vi "Interpret ADS Packet.vi"(8 "Error In":errorcluster, 11 "ADS Packet":string) -> (0 "Error Out":errorcluster, 2 "AMS":T1, 3 "Data":u8[](array[numeric]), 4 "Invoke ID":u32, 5 "State Flag":T3=4 items=["TCP Request"=4, "TCP Response"=5, "UDP Request"=68, "UDP Respone"=69], 6 "ADS Error":T2 items=["NoError"=0, "InternalError"=1, "NoRTime"=2, "LockedMemoryError"=3, "MailBoxError"=4, "WrongHMsg"=5, "TargetPortNotFound"=6, "TargetMachineNotFound"=7, "UnknownCommandID"=8, "BadTaskID"=9, "NoIO"=10, "UnknownAmsCommand"=11, "Win32Error"=12, "PortNotConnected"=13, "InvalidAmsLength"=14, "InvalidAmsNetID"=15, "AmsSyncAmsError"=22, "AmsSyncNoIndexMap"=23, "InvalidAmsPort"=24, "NoMemory"=25, "TCPSendError"=26, "HostUnreachable"=27, "NoLockedMemory"=1280, "MailboxFull"=1282, "DeviceError"=1792, "DeviceServiceNotSupported"=1793, "DeviceInvalidGroup"=1794, "DeviceInvalidOffset"=1795, "DeviceInvalidAccess"=1796, "DeviceInvalidSize"=1797, "DeviceInvalidData"=1798, "DeviceNotReady"=1799, "DeviceBusy"=1800, "DeviceInvalidContext"=1801, "DeviceNoMemory"=1802, "DeviceInvalidParam"=1803, "DeviceNotFound"=1804, "DeviceSyntaxError"=1805, "DeviceIncompatible"=1806, "DeviceExists"=1807, "DeviceSymbolNotFound"=1808, "DeviceSymbolVersionInvalid"=1809, "DeviceInvalidState"=1810, "DeviceTransModeNotSupported"=1811, "DeviceNotifyHandleInvalid"=1812, "DeviceClientUnknown"=1813, "DeviceNoMoreHandles"=1814, "DeviceInvalidWatchsize"=1815, "DeviceNotInitialized"=1816, "DeviceTimeOut"=1817, "DeviceNoInterface"=1818, "DeviceInvalidInterface"=1819, "DeviceInvalidCLSID"=1820, "DeviceInvalidObjectID"=1821, "ClientError"=1856, "ClientInvalidParameter"=1857, "ClientListEmpty"=1858, "ClientVariableInUse"=1859, "ClientDuplicateInvokeID"=1860, "ClientSyncTimeOut"=1861, "ClientW32OR"=1862, "ClientTimeoutInvalid"=1863, "ClientPortNotOpen"=1864, "ClientNoAmsAddr"=1865, "ClientSyncInternal"=1872, "ClientAddHash"=1873, "ClientRemoveHash"=1874, "ClientNoMoreSymbols"=1875, "ClientSyncResInvalid"=1876, "ClientSyncPortLocked"=1877, "ClientQueueFull"=1878], 7 "Command ID":T4=enum."ADS Read Device Info")   [LabVIEW 2019, in "TwinCAT ADS.lvlib"]
uses:
  <userlib>/PMA/TwinCAT ADS.lvlib
  <userlib>/PMA/Low Level/TypeDefs/Command Id.ctl
  <userlib>/PMA/Low Level/TypeDefs/State Flag.ctl
  <userlib>/PMA/Low Level/TypeDefs/ADS Error.ctl
  <userlib>/PMA/Low Level/TypeDefs/AMS.ctl
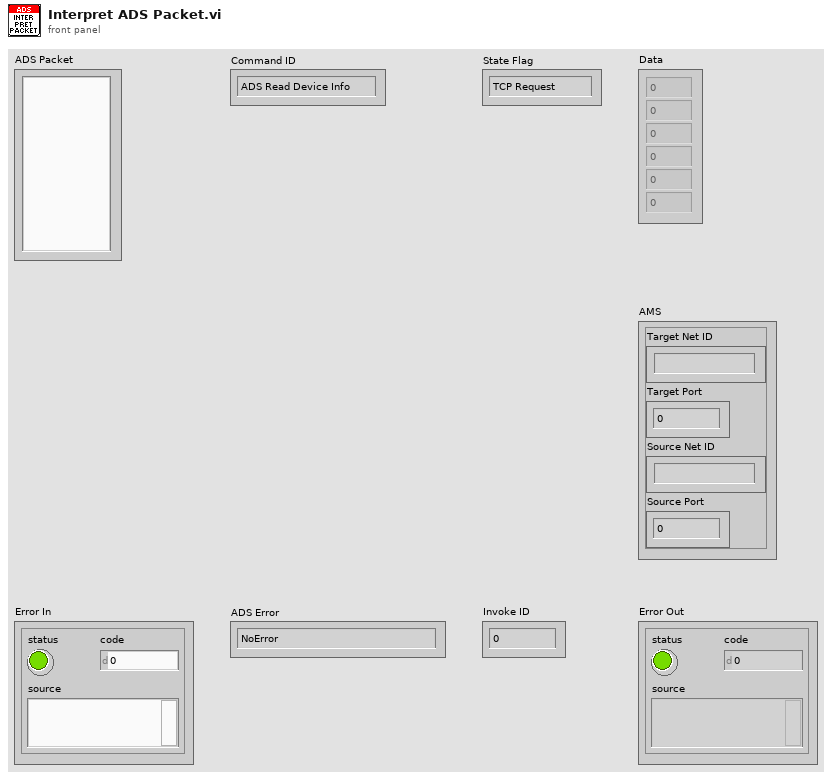
[diagram p1: front panel]
types:
  T1 = typedef "TwinCAT ADS.lvlib/AMS.ctl" = cluster{"Target Net ID":string, "Target Port":u16, "Source Net ID":string, "Source Port":u16}
  T2 = typedef "TwinCAT ADS.lvlib/ADS Error.ctl" = i32
  T3 = typedef "TwinCAT ADS.lvlib/State Flag.ctl" = u16
  T4 = typedef "TwinCAT ADS.lvlib/Command Id.ctl" = enum16{"Invalid", "ADS Read Device Info", "ADS Read", "ADS Write", "ADS Read State", "ADS Write Control", "ADS Add Device Notification", "ADS Delete Device Notification", "ADS Device Notification", "ADS Read Write"}
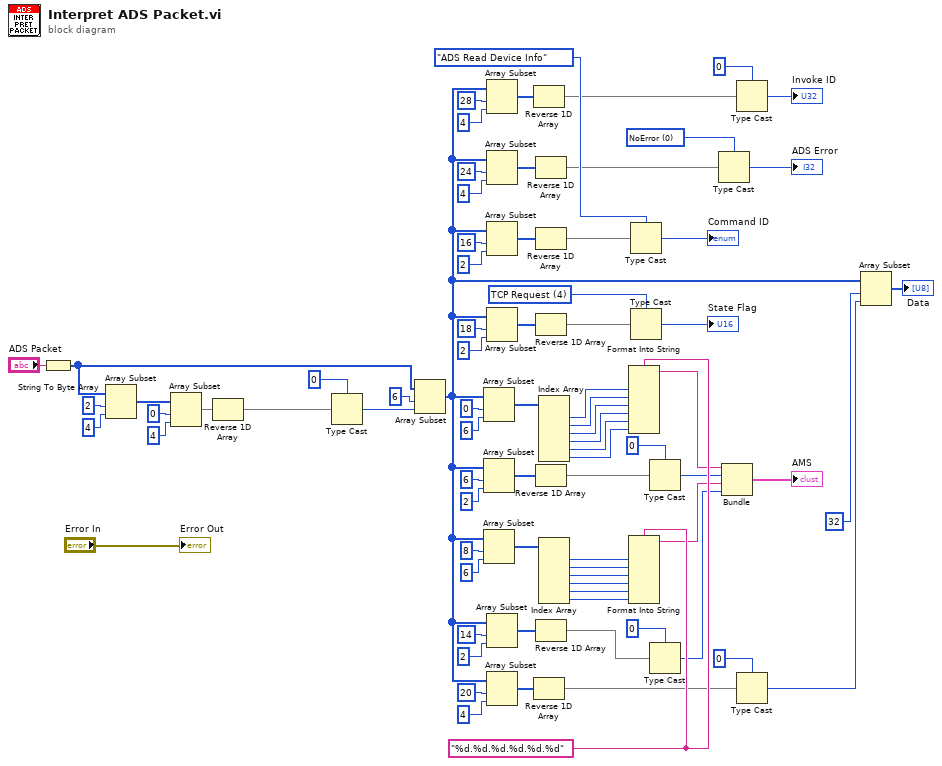
[diagram p0: block diagram]
diagram:
  w16 = T2 0 items=["NoError"=0, "InternalError"=1, "NoRTime"=2, "LockedMemoryError"=3, "MailBoxError"=4, "WrongHMsg"=5, "TargetPortNotFound"=6, "TargetMachineNotFound"=7, "UnknownCommandID"=8, "BadTaskID"=9, "NoIO"=10, "UnknownAmsCommand"=11, "Win32Error"=12, "PortNotConnected"=13, "InvalidAmsLength"=14, "InvalidAmsNetID"=15, "AmsSyncAmsError"=22, "AmsSyncNoIndexMap"=23, "InvalidAmsPort"=24, "NoMemory"=25, "TCPSendError"=26, "HostUnreachable"=27, "NoLockedMemory"=1280, "MailboxFull"=1282, "DeviceError"=1792, "DeviceServiceNotSupported"=1793, "DeviceInvalidGroup"=1794, "DeviceInvalidOffset"=1795, "DeviceInvalidAccess"=1796, "DeviceInvalidSize"=1797, "DeviceInvalidData"=1798, "DeviceNotReady"=1799, "DeviceBusy"=1800, "DeviceInvalidContext"=1801, "DeviceNoMemory"=1802, "DeviceInvalidParam"=1803, "DeviceNotFound"=1804, "DeviceSyntaxError"=1805, "DeviceIncompatible"=1806, "DeviceExists"=1807, "DeviceSymbolNotFound"=1808, "DeviceSymbolVersionInvalid"=1809, "DeviceInvalidState"=1810, "DeviceTransModeNotSupported"=1811, "DeviceNotifyHandleInvalid"=1812, "DeviceClientUnknown"=1813, "DeviceNoMoreHandles"=1814, "DeviceInvalidWatchsize"=1815, "DeviceNotInitialized"=1816, "DeviceTimeOut"=1817, "DeviceNoInterface"=1818, "DeviceInvalidInterface"=1819, "DeviceInvalidCLSID"=1820, "DeviceInvalidObjectID"=1821, "ClientError"=1856, "ClientInvalidParameter"=1857, "ClientListEmpty"=1858, "ClientVariableInUse"=1859, "ClientDuplicateInvokeID"=1860, "ClientSyncTimeOut"=1861, "ClientW32OR"=1862, "ClientTimeoutInvalid"=1863, "ClientPortNotOpen"=1864, "ClientNoAmsAddr"=1865, "ClientSyncInternal"=1872, "ClientAddHash"=1873, "ClientRemoveHash"=1874, "ClientNoMoreSymbols"=1875, "ClientSyncResInvalid"=1876, "ClientSyncPortLocked"=1877, "ClientQueueFull"=1878] ("Enum")
  w29 = T3 4 items=["TCP Request"=4, "TCP Response"=5, "UDP Request"=68, "UDP Respone"=69] ("State Flag")
  w46 = "%d.%d.%d.%d.%d.%d" ("format string")
  n1 = String To Byte Array(string="ADS Packet") -> (unsigned byte array=w1:u8[])
  n2 = Array Subset(array=w1, index=2, length=4) -> (w63:u8[])
  n3 = Array Subset(array=w63, index=0, length=4) -> (w77:u8[])
  n4 = Reverse 1D Array(array=w77) -> (reversed array=w75:u8[])
  n5 = Type Cast(type=u32 0, x=w75) -> (*(type *) &x=w74:u32)
  n6 = Array Subset(array=w1, index=6, length=w74) -> (w10:u8[])
  n7 = Array Subset(array=w10, index=0, length=6) -> (w70:u8[])
  n8 = Array Subset(array=w10, index=6, length=2) -> (w60:u8[])
  n9 = Array Subset(array=w10, index=8, length=6) -> (w49:u8[])
  n10 = Array Subset(array=w10, index=28, length=4) -> (w13:u8[])
  n11 = Array Subset(array=w10, index=24, length=4) -> (w20:u8[])
  n12 = Array Subset(array=w10, index=16, length=2) -> (w38:u8[])
  n13 = Array Subset(array=w10, index=18, length=2) -> (w33:u8[])
  n14 = Array Subset(array=w10, index=14, length=2 ("index")) -> (w43:u8[])
  n15 = Array Subset(array=w10, index=20, length=4) -> (w26:u8[])
  n16 = Reverse 1D Array(array=w13) -> (reversed array=w14:u8[])
  n17 = Reverse 1D Array(array=w26) -> (reversed array=w25:u8[])
  n18 = Reverse 1D Array(array=w20) -> (reversed array=w17:u8[])
  n19 = Reverse 1D Array(array=w38) -> (reversed array=w35:u8[])
  n20 = Reverse 1D Array(array=w33) -> (reversed array=w34:u8[])
  n21 = Reverse 1D Array(array=w60) -> (reversed array=w59:u8[])
  n22 = Reverse 1D Array(array=w43) -> (reversed array=w44:u8[])
  n23 = Index Array(array=w70) -> (element #1=w69:u8, element #2=w68:u8, element #3=w67:u8, element #4=w66:u8, element #5=w65:u8, element #6=w64:u8)  [unwired: 6 in]
  n24 = Index Array(array=w49) -> (element #1=w50:u8, element #2=w51:u8, element #3=w52:u8, element #4=w53:u8, element #5=w54:u8, element #6=w55:u8)  [unwired: 6 in]
  n25 = Format Into String(format string=w46, w69, w68, w67, w66, w65, w64) -> (resulting string=w7:string)  [unwired: 2 in, 1 out]
  n26 = Format Into String(format string=w46, w50, w51, w52, w53, w54, w55) -> (resulting string=w4:string)  [unwired: 2 in, 1 out]
  n27 = Type Cast(type=Command_Id."ADS Read Device Info" ("Command ID"), x=w35) -> (*(type *) &x=→"Command ID":T4)
  n28 = Type Cast(type=w29, x=w34) -> (*(type *) &x=→"State Flag":T3)
  n29 = Type Cast(type=u16 0, x=w59) -> (*(type *) &x=w5:u16)
  n30 = Type Cast(type=u16 0, x=w44) -> (*(type *) &x=w6:u16)
  n31 = Type Cast(type=w16, x=w17) -> (*(type *) &x=→"ADS Error":T2)
  n32 = Bundle(w7, w5, w4, w6) -> (→"AMS":cluster{string, u16, string, u16})  [unwired: 1 in]
  n33 = Type Cast(type=u32 0 ("Invoke ID"), x=w14) -> (*(type *) &x=→"Invoke ID":u32)
  n34 = Type Cast(type=u32 0, x=w25) -> (*(type *) &x=w23:u32)
  n35 = Array Subset(array=w10, index=32, length=w23) -> (→"Data":u8[])
  "Error Out" <- "Error In"
